vi "UpdateFailbar.vi"(9 "Progress":u32, 10 "Function":T1=enum."Update Progress", 11 "Slide Refnum":refnum<vi>) -> ()   [LabVIEW 2011, in "GraphicalTestRunner.lvlib"]
uses:
  GraphicalTestRunner.lvlib
  FailbarStatus--Enum.ctl
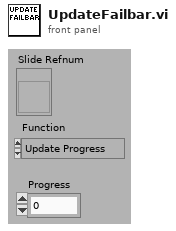
[diagram p1: front panel]
types:
  T1 = typedef "GraphicalTestRunner.lvlib/FailbarStatus--Enum.ctl" = enum16{"Initialize", "Start", "Update Progress", "Fail", "Pass"}
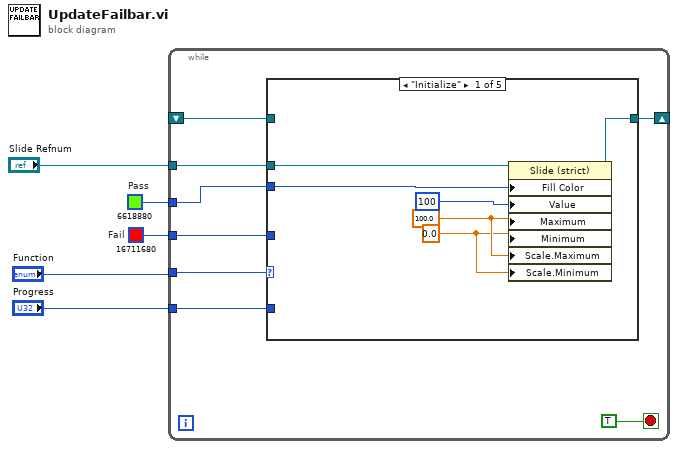
[diagram p0: block diagram]
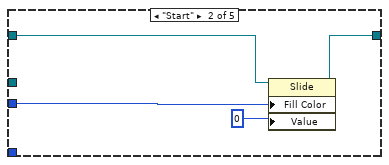
[diagram p2: hidden frame]
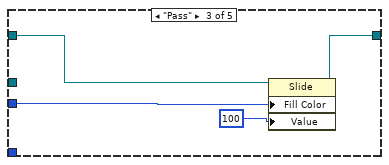
[diagram p3: hidden frame]
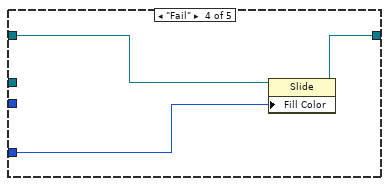
[diagram p4: hidden frame]
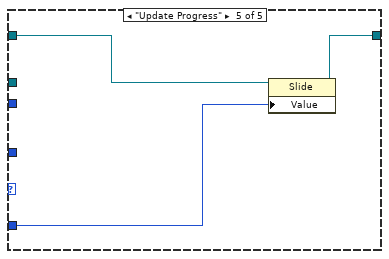
[diagram p5: hidden frame]
diagram:
  w3 = u32 6618880  # Pass
  w1 = u32 16711680  # Fail
  n1 = while {
    tunnel: "Slide Refnum" -> [w13]
    tunnel: "Function" -> [w11]
    tunnel: w3 -> [w10]
    tunnel: "Progress" -> [w9]
    tunnel: w1 -> [w8]
    shift-right: [w7] -> _
    shift-left: _ -> [w6]
    stop <- TRUE stop-if-true
    n2 = case shown="\"Initialize\"" w11 {
      tunnel: w13 -> [w19 _ _ _ _]
      tunnel: w10 -> [w18 w23 w27 _ _]
      tunnel: w9 -> [_ _ _ _ w33]
      tunnel: w8 -> [_ _ _ w30 _]
      tunnel: [w16 w21 w25 w28 w31] -> w7
      tunnel: w6 -> [_ w20 w24 w29 w32]
      frame "Initialize" {
        w14 = 0.0 ("Data Range:Minimum")
        w15 = 100.0 ("Data Range:Maximum")
        n3 = property on="Property Node" class="Slide (strict)"(reference=w19, "Fill Color"=w18, "Value"=u8 100, "Maximum"=w15, "Minimum"=w14, "Scale.Maximum"=w15, "Scale.Minimum"=w14) -> (reference out=w16:refnum<vi>)  [unwired: 1 in, 1 out]
      }
      frame "Start" {
        n4 = property on="Property Node" class="Slide"(reference=w20, "Fill Color"=w23, "Value"=u8 0) -> (reference out=w21:refnum<vi>)  [unwired: 1 in, 1 out]
      }
      frame "Pass" {
        n5 = property on="Property Node" class="Slide"(reference=w24, "Fill Color"=w27, "Value"=u8 100) -> (reference out=w25:refnum<vi>)  [unwired: 1 in, 1 out]
      }
      frame "Fail" {
        n6 = property on="Property Node" class="Slide"(reference=w29, "Fill Color"=w30) -> (reference out=w28:refnum<vi>)  [unwired: 1 in, 1 out]
      }
      frame "Update Progress" {
        n7 = property on="Property Node" class="Slide"(reference=w32, "Value"=w33) -> (reference out=w31:refnum<vi>)  [unwired: 1 in, 1 out]
      }
    }
  }
